vi "test1.vi"() -> ()   [LabVIEW 2019]
panel:
  in  "Next":bool
  in  "autoMove":bool
  in  "y0":dbl(slide) scale=-115.0..115.0
  in  "z0":dbl(slide) scale=-135.0..50.0
  in  "x0":dbl(slide) scale=-115.0..115.0
  in  "clip":dbl(slide)=15.0 scale=0.0..15.0
  in  "turn":dbl(knob) scale=-150.0..110.0
  out "turnout":dbl
  in  "stop":bool
  in  "move to":T1(ring)=enum."P3"
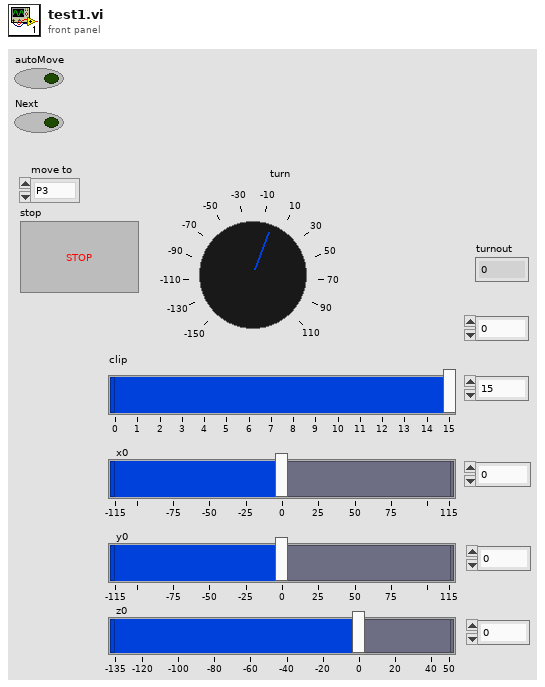
[diagram p1: front panel]
types:
  T1 = enum16{"P1", "P2", "P3", "P4", "P5", "P6", "OUT"}
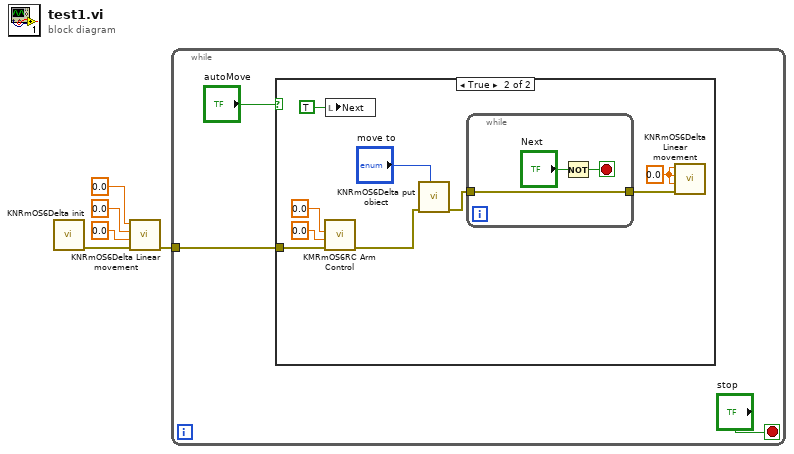
[diagram p0: block diagram]
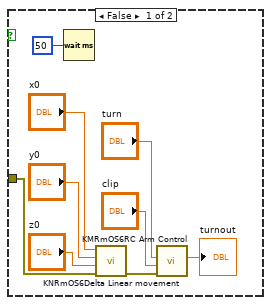
[diagram p2: hidden frame]
diagram:
  n1 = call "KNRmOS6Delta init.vi"() -> ("error out"=w2:errorcluster)  [unwired: 11 in]
  n2 = call "KNRmOS6Delta Linear movement.vi"("error in (no error)"=w2, "z0"=0.0, "y0"=0.0, "x0"=0.0) -> ("error out"=w1:errorcluster)  [unwired: 7 in]
  n3 = while {
    tunnel: w1 -> [w7]
    stop <- "stop" stop-if-true
    n4 = case shown="True" "autoMove" {
      tunnel: w7 -> [w14 w22]
      frame False {
        n5 = Wait (ms)(milliseconds to wait=u32 50) -> ()  [unwired: 1 out]
        n6 = call "KNRmOS6Delta Linear movement.vi"("error in (no error)"=w14, "z0"="z0", "y0"="y0", "x0"="x0") -> ("error out"=w13:errorcluster)  [unwired: 7 in]
        n7 = call "KMRmOS6RC Arm Control.vi"("error in (no error)"=w13, "clip"="clip", "turn"="turn") -> ("turnout"=→"turnout":dbl)  [unwired: 6 in, 2 out]
      }
      frame True {
        w18 = 0.0 ("x0")
        n8 = call "KMRmOS6RC Arm Control.vi"("error in (no error)"=w22, "clip"=0.0, "turn"=0.0) -> ("error out"=w25:errorcluster)  [unwired: 6 in, 2 out]
        n9 = local write "Next"(TRUE ("Next")) -> ()
        n10 = call "KNRmOS6Delta put obiect.vi"("move to"="move to", "error in (no error)"=w25) -> ("error in (no error) 2"=w21:errorcluster)  [unwired: 9 in]
        n11 = while {
          tunnel: w21 -> [w27]
          tunnel: [w27] -> w19
          stop <- w28 stop-if-true
          n12 = Not(x="Next") -> (.not. x?=w28:bool)
        }
        n13 = call "KNRmOS6Delta Linear movement.vi"("error in (no error)"=w19, "z0"=w18, "y0"=w18, "x0"=w18) -> ()  [unwired: 7 in, 1 out]
      }
    }
  }
